vi "RFID Details.vi"(8 "error in (no error)":errorcluster, 10 "RFID":string, 11 "Ref In":T1={"MS SQL Connection"=refnum, "UDL File"=path "", "Time"="", "DCODE"="", "WIP+1"=0, "MC No?"=0, "POKAYOKE?"=FALSE, "Expected Result"="", "Result [Status]"="", "Clock"=0.0, "RFID"="", "WIP Queue"=refnum, "TS Parameter"={"ProfitCenterCode"="", "LineCode"="", "WorkOrderNumber"="", "Model"="", "Model_with_Prefix"="", "VendorCode"="", "SetParameterDateCode"="", "PokaYoke"=0, "Target"=1, "Live_DateCode"="", "CustomerPartNumber"="", "Hand"="", "Ent_Stamp"=timestamp(0 s since 1904-01-01), "sBarcode"=FALSE, "FCA"=0, "STS_CD"=0.0}, "Data_Queue"=[], "RFID Serial No."=""} {"TS Parameter"."FCA" format="%01d"; "TS Parameter"."Target" min=1 max=100000; "TS Parameter"."PokaYoke" min=0 max=1}) -> (0 "error out":errorcluster, 2 "Header":string[](array[string]), 3 "Data":string[][](array[string]))   [LabVIEW 2020]
uses:
  Controls/TD SQL.ctl
  <vilib>/addons/database/Connection.llb/Conn ObjectReference.ctl
  Controls/WIP_State.ctl
  Controls/TS_Parameter.ctl
  MS SQL/MS_Global.vi
  <vilib>/addons/database/NI_Database_API.lvlib
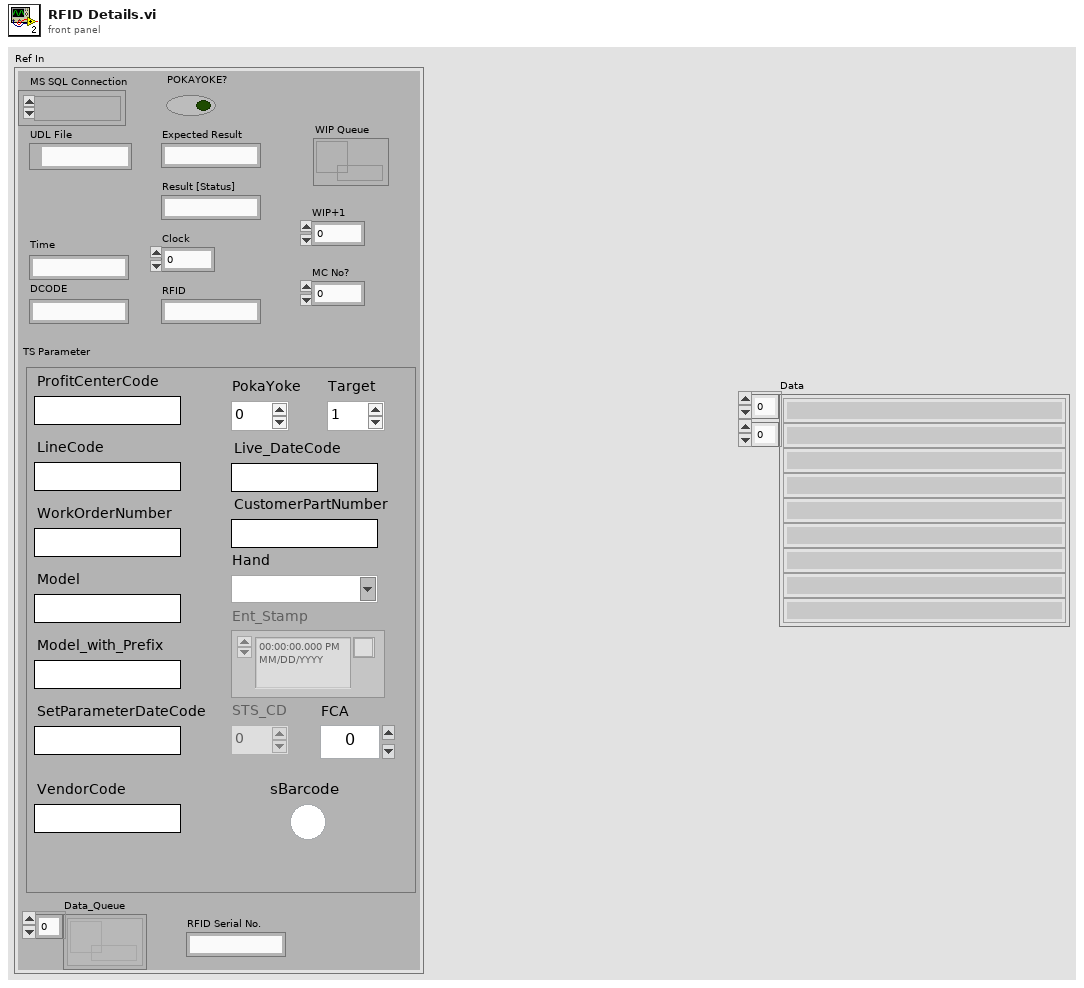
[diagram p1: front panel]
types:
  T1 = typedef "TD SQL.ctl" = cluster{"MS SQL Connection":T2, "UDL File":path, "Time":string, "DCODE":string, "WIP+1":i64, "MC No?":i32, "POKAYOKE?":bool, "Expected Result":string, "Result [Status]":string, "Clock":dbl, "RFID":string, "WIP Queue":refnum<queue>, "TS Parameter":T3, "Data_Queue":refnum<queue>[], "RFID Serial No.":string}
  T2 = typedef "NI_Database_API.lvlib/Conn ObjectReference.ctl" = refnum<k1>
  T3 = typedef "TS_Parameter.ctl" = cluster{"ProfitCenterCode":string, "LineCode":string, "WorkOrderNumber":string, "Model":string, "Model_with_Prefix":string, "VendorCode":string, "SetParameterDateCode":string, "PokaYoke":i32, "Target":i32, "Live_DateCode":string, "CustomerPartNumber":string, "Hand":string, "Ent_Stamp":timestamp, "sBarcode":bool, "FCA":i32, "STS_CD":dbl}
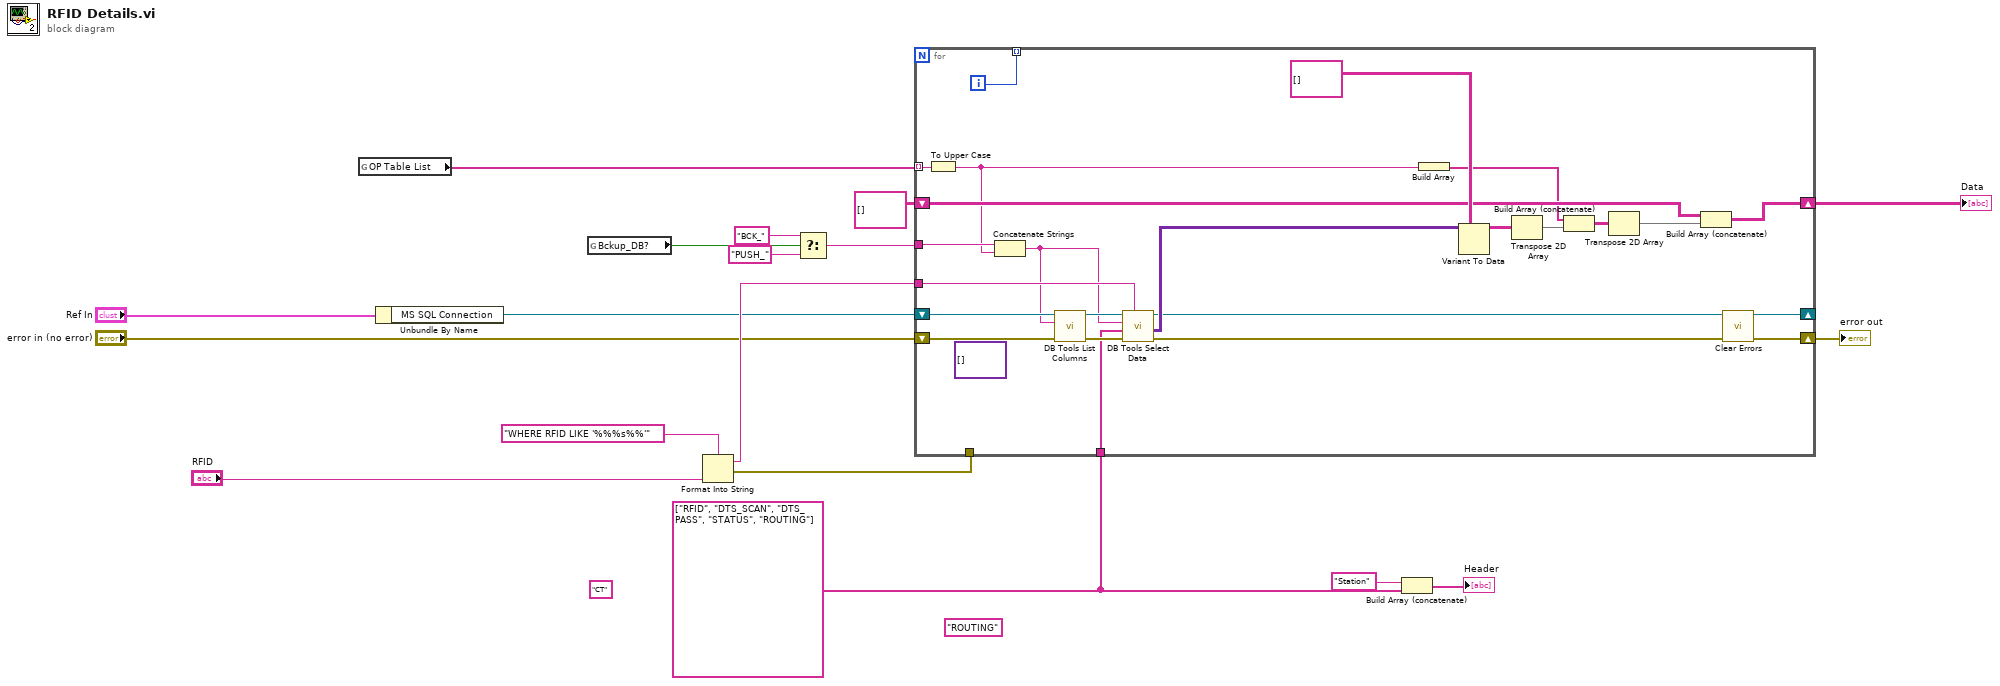
[diagram p0: block diagram]
diagram:
  (unwired) "ROUTING" ("String")
  (unwired) "CT" ("String")
  w16 = string[] ["RFID", "DTS_SCAN", "DTS_PASS", "STATUS", "ROUTING"] ("columns")
  n1 = global read "MS_Global.vi" "OP Table List"() -> (w5:string[])
  n2 = Unbundle By Name("Ref In") -> ("MS SQL Connection"=w8:T2)
  n3 = global read "MS_Global.vi" "Bckup_DB?"() -> (w2:bool)
  n4 = Format Into String(format string="WHERE RFID LIKE '%%%s%%'" ("condition"), "RFID") -> (resulting string=w12:string, error out=w13:errorcluster)  [unwired: 2 in]
  n5 = Select(t="BCK_", s=w2, f="PUSH_") -> (s? t:f=w1:string)
  n6 = for {
    tunnel: w5 -> [w24] mode=indexing
    shift-right: [w41] -> w15
    shift-left: "error in (no error)" -> [w37]
    shift-right: [w30] -> _
    shift-left: w8 -> [w38]
    tunnel: w16 -> [w19]
    shift-right: [w31] -> w14
    shift-left: string[][] [] -> [w32]
    tunnel: w12 -> [w28]
    tunnel: w13 -> [_]
    tunnel: [w23] -> _ mode=indexing
    tunnel: w1 -> [w22]
    i -> [w23]
    (unwired) variant[][] [] ("data")
    n7 = To Upper Case(1:w24) -> (0:w20:string)
    n8 = Concatenate Strings(w22, w20) -> (w21:string)
    n9 = call <vilib>:"DB Tools List Columns.vi"("error in (no error)"=w37, "table"=w21, "connection reference"=w38) -> ("error out"=w40:errorcluster, "connection reference out"=w39:T2)  [unwired: 1 in, 2 out]
    n10 = call <vilib>:"DB Tools Select Data.vi"("condition"=w28, "error in (no error)"=w40, "columns"=w19, "table"=w21, "connection reference"=w39) -> ("error out"=w29:errorcluster, "data"=w36:variant[][], "connection reference out"=w30:T2)  [unwired: 1 in]
    n11 = Build Array(w20) -> (w27:string[])
    n12 = Variant To Data(type=string[][] [] ("columns"), Variant=w36) -> (data=w34:string[][])  [unwired: 1 in, 1 out]
    n13 = Transpose 2D Array(2D array=w34) -> (transposed array=w26:string[][])
    n14 = Build Array (concatenate)(w27, w26) -> (w33:string[][])
    n15 = Transpose 2D Array(2D array=w33) -> (transposed array=w25:string[][])
    n16 = Build Array (concatenate)(w32, w25) -> (w31:string[][])
    n17 = call <vilib>:"Clear Errors.vi"("error in (no error)"=w29) -> ("error out"=w41:errorcluster)  [unwired: 5 in, 1 out]
  }
  "error out" <- w15
  "Data" <- w14
  n18 = Build Array (concatenate)("Station" ("String"), w16) -> (→"Header":string[])
